vi "读取表格多个sheet数据并分类.vi"(7 "错误 in":errorcluster caption="错误常量", 8 "各sheet名称数组":string[](array[string]), 11 "File in":path) -> (1 "Cam1Light1数据":string[][](array[string]), 3 "存储数据 2":cluster{"Cam1Light1数据":string[][]})   [LabVIEW 2014]
panel:
  out "data":string[][](array[string])
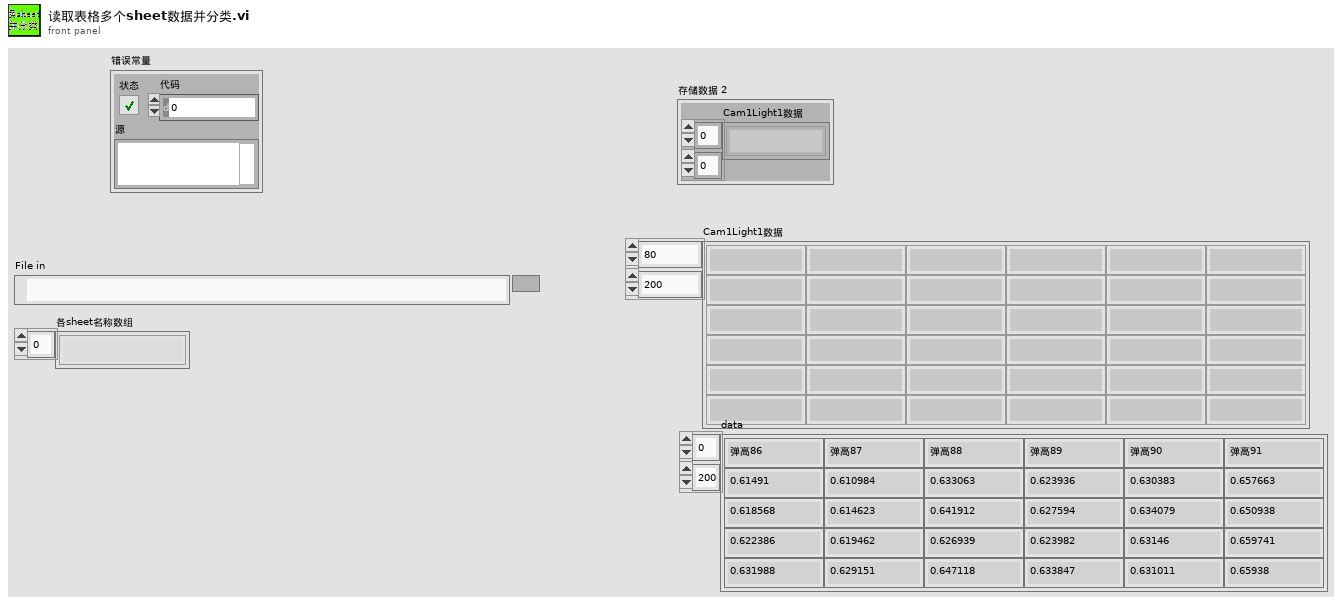
[diagram p1: front panel]
types:
  T1 = typedef "控件-Excel读写选项.ctl" = enum16{"打开表格", "新增sheet", "读取sheet指定位置数据", "读取sheet整个数据", "写入sheet整个数据", "写表头", "数据存到本机", "表格是否开启状态", "关闭表格"}
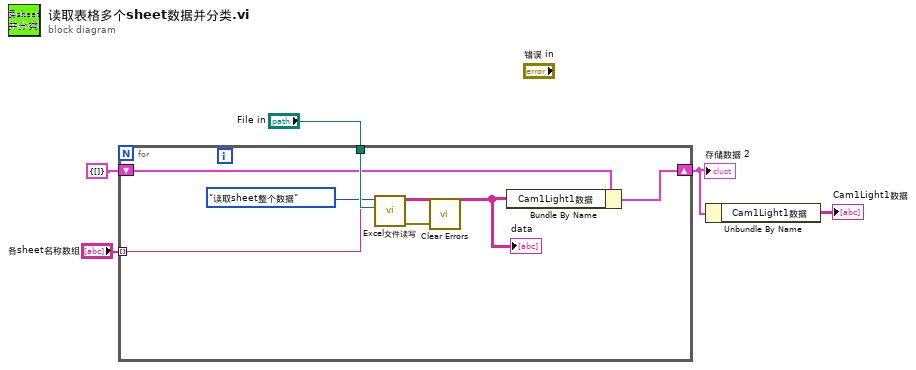
[diagram p0: block diagram]
diagram:
  n1 = for {
    tunnel: "File in" -> [w12]
    tunnel: "各sheet名称数组" -> [w11] mode=indexing
    shift-right: [w9] -> w2
    shift-left: cluster{"Cam1Light1数据":string[][]} {"Cam1Light1数据"=[]} ("存储数据 2") -> [w10]
    n2 = call "Excel文件读写.vi"("Path"=w12, "worksheet name"=w11, "选项"=控件-Excel读写选项."读取sheet整个数据") -> ("error out"=w8:errorcluster, "data"=w7:string[][])  [unwired: 4 in, 1 out]
    "data" <- w7
    n3 = call <vilib>:"Clear Errors.vi"("error in (no error)"=w8) -> ()  [unwired: 5 in, 2 out]
    n4 = Bundle By Name(cluster=w10, "Cam1Light1数据"=w7) -> (w9:cluster{"Cam1Light1数据":string[][]})
  }
  "存储数据 2" <- w2
  n5 = Unbundle By Name(w2) -> ("Cam1Light1数据"=→"Cam1Light1数据":string[][])
